vi "Disconnect from Target.vi"(8 "error in (no error)":errorcluster, 11 "SV B-M (Host) in":refnum<class "SV B-M (Host).lvclass">) -> (0 "error out":errorcluster, 3 "SV B-M (Host) out":refnum<class "SV B-M (Host).lvclass">)   [LabVIEW 2015, in "SV B-M (Host).lvclass"]
doc: "Disconnect from target by destroying command & ack network streams."
uses:
  SV B-M (Host).lvclass
  Listbox - In Progress.vi
  Command & Ack - Destroy Endpoints.vi
  Listbox - Complete.vi
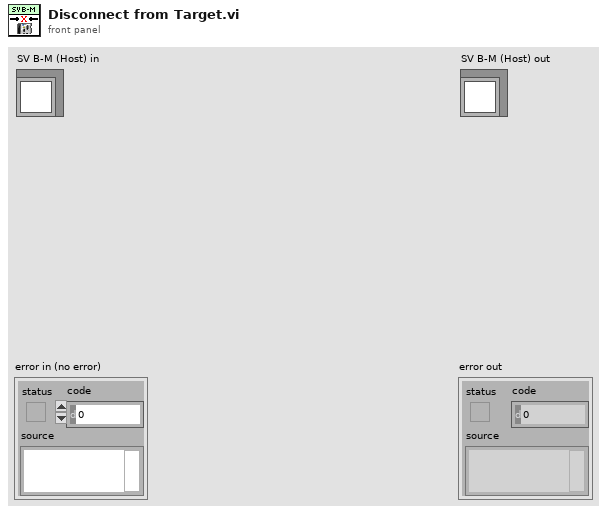
[diagram p1: front panel]
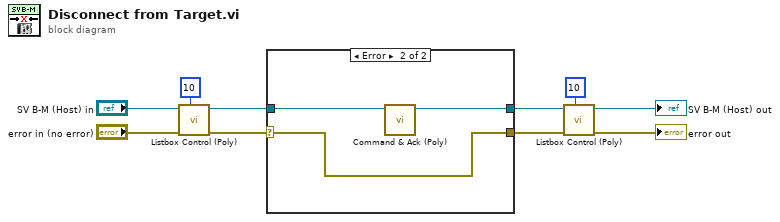
[diagram p0: block diagram]
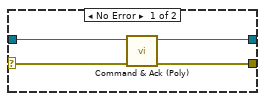
[diagram p2: hidden frame]
diagram:
  n1 = call-poly "Listbox Control (Poly).vi"("Row to Update"=10, "error in (no error)"="error in (no error)", "SV B-M In"="SV B-M (Host) in") -> ("error out"=w4:errorcluster, "SV B-M Out"=w5:refnum<class "SV B-M (Host).lvclass">)  [unwired: 7 in]
  n2 = case shown="Error" w4 {
    selector: w4 -> [w12 w15]
    tunnel: [w11 w15] -> w3
    tunnel: [w13 w16] -> w6
    tunnel: w5 -> [w14 w17]
    frame No Error {
      n3 = call-poly "Command & Ack (Poly).vi"("error in (no error)"=w12, "SV B-M (Host) in"=w14) -> ("error out"=w11:errorcluster, "SV B-M (Host) out"=w13:refnum<class "SV B-M (Host).lvclass">)  [unwired: 8 in]
    }
    frame Error {
      n4 = call-poly "Command & Ack (Poly).vi"("SV B-M (Host) in"=w17) -> ("SV B-M (Host) out"=w16:refnum<class "SV B-M (Host).lvclass">)  [unwired: 9 in, 1 out]
    }
  }
  n5 = call-poly "Listbox Control (Poly).vi"("Row to Update"=10, "error in (no error)"=w3, "SV B-M In"=w6) -> ("error out"=→"error out":errorcluster, "SV B-M Out"=→"SV B-M (Host) out":refnum<class "SV B-M (Host).lvclass">)  [unwired: 7 in]
